vi "Board Adjustment.vi"(4 "DAC Value":u32=32768, 5 "DAC Ch#":i32=7, 6 "Board":T1 items=["Quad DC Board", "Lens 1 (Slot 8) Module", "Lens 2 (Slot 6) Module", "Detector Board", "Quad DC Board with Test Points", "Lens 1 Module with Test Points", "Len 2 Module with Test Points", "", "", "", "", ""], 7 "Test Points":string="Q1A and Q1B", 8 "DAC Channel Name":string="Q1 Resolution DC (Q1 RR)") -> (3 "Final DAC":u32)   [LabVIEW 2012]
uses:
  Type/_Board ID.ctl
  Configuration/_Global Configuration.vi
panel:
  in  "Done":bool
  # "Please attach test leads from your DVM to specified test points indicated below.\nAdjust the DAC Value manually until the reading is 0 VDC.\nClick Done when complete."
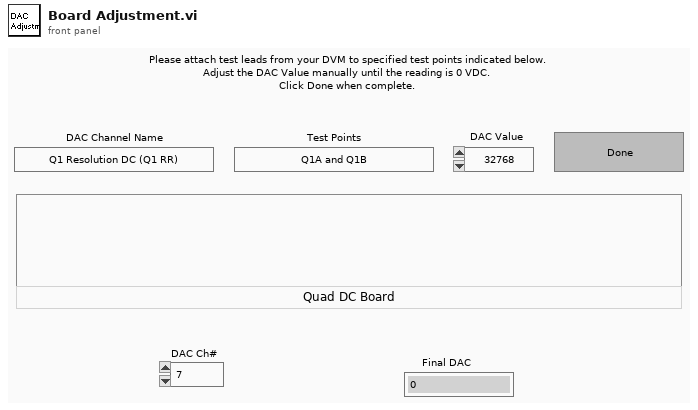
[diagram p1: front panel]
types:
  T1 = typedef "_Board ID.ctl" = u16
  T2 = typedef "_RT Instrument 2.ctl" = cluster{"Table":T3[], "Instrument":string[]}
  T3 = typedef "_RT Configuration 2.ctl" = cluster{"Name":string, "Ch#":u8, "Min":dbl, "Max":dbl, "Def+":dbl, "Def-":dbl, "Offset":dbl, "Slope":dbl, "Type":u8, "Description":string, "SettleT":dbl}
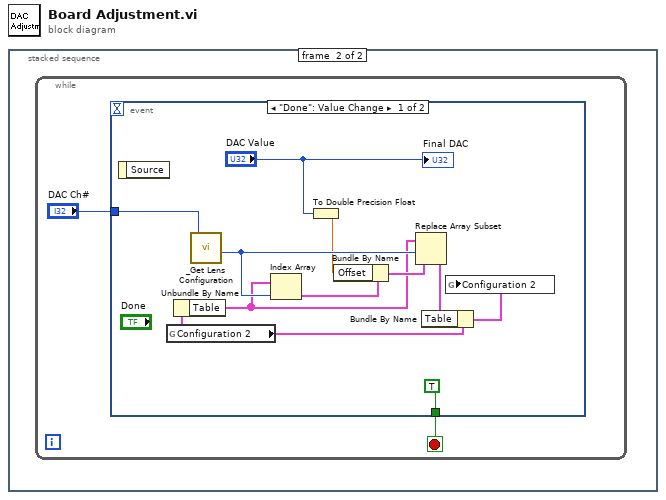
[diagram p0: block diagram]
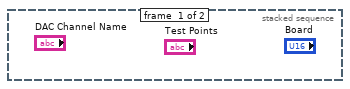
[diagram p2: hidden frame]
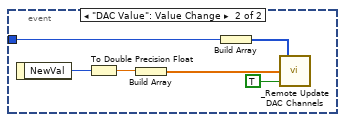
[diagram p3: hidden frame]
diagram:
  n1 = stacked-sequence {
    frame #0 {
    }
    frame #1 {
      n2 = while {
        stop <- w2 stop-if-true
        n3 = event shown="[0] \"Done\": Value Change" {
          selector: _ -> [_ _]
          dyn-events: _ -> [_ _]
          timeout: _ -> [_ _]
          tunnel: [TRUE _] -> w2
          tunnel: "DAC Ch#" -> [w5 w14]
          event "Done": Value Change {
            n4 = event-data() -> ()  [unwired: 2 out]
            n5 = global read "_Global Configuration.vi" "Configuration 2"() -> (w7:T2)
            n6 = Unbundle By Name(w7) -> ("Table"=w9:T3[])
            n7 = call "_Get Lens Configuration.vi"("Channel #"=w5) -> ("Config Row#"=w11:i32)  [unwired: 1 in, 5 out]
            n8 = Index Array(array=w9, index=w11) -> (element=w12:T3)
            n9 = To Double Precision Float(number="DAC Value") -> (double precision float=w3:dbl)
            n10 = Bundle By Name(cluster=w12, "Offset"=w3) -> (w10:T3)
            n11 = Replace Array Subset(array=w9, new element=w10, index=w11) -> (w8:T3[])
            n12 = Bundle By Name(cluster=w7, "Table"=w8) -> (w6:T2)
            n13 = global write "_Global Configuration.vi" "Configuration 2"(w6) -> ()
            "Final DAC" <- "DAC Value"
          }
          event "DAC Value": Value Change {
            n14 = event-data() -> ("NewVal"=w17:u32)  [unwired: 1 out]
            n15 = To Double Precision Float(number=w17) -> (double precision float=w16:dbl)
            n16 = Build Array(w16) -> (w15:dbl[])
            n17 = Build Array(w14) -> (w19:i32[])
            n18 = call "_Remote Update DAC Channels.vi"("In DAC(F)"=TRUE, "UserValue"=w15, "Ch#"=w19) -> ()  [unwired: 2 out]
          }
        }
      }
    }
  }
